vi "Write Value.vi"(8 "error in (no error)":errorcluster, 10 "Value":bool, 11 "Boolean Parameter in":refnum<class "Boolean Parameter.lvclass">) -> (0 "error out":errorcluster, 3 "Boolean Parameter out":refnum<class "Boolean Parameter.lvclass">)   [LabVIEW 2019, in "CD Parameter Manager API.lvlib" / "Boolean Parameter.lvclass"]
uses:
  Boolean Parameter.lvclass
  Boolean Parameter.lvclass/Boolean Parameter.ctl
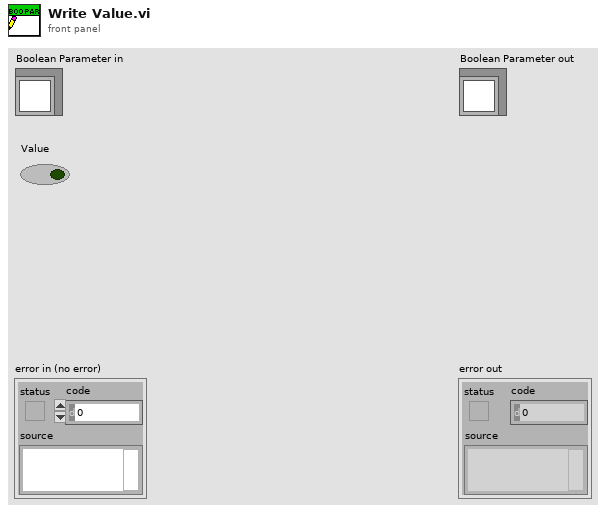
[diagram p1: front panel]
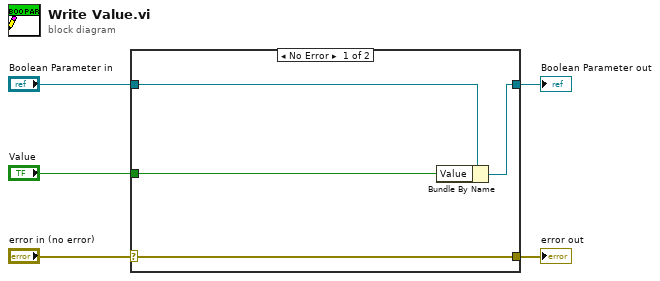
[diagram p0: block diagram]
diagram:
  n1 = case shown="No Error" "error in (no error)" {
    selector: "error in (no error)" -> [w9 w10]
    tunnel: [w9 w10] -> w4
    tunnel: [w7 w11] -> w2
    tunnel: "Boolean Parameter in" -> [w8 w11]
    tunnel: "Value" -> [w6 _]
    frame No Error {
      n2 = Bundle By Name(cluster=w8, "Value"=w6) -> (w7:refnum<class "Boolean Parameter.lvclass">)
    }
    frame Error {
    }
  }
  "error out" <- w4
  "Boolean Parameter out" <- w2
